vi "DWDT Digital to Binary U32.vi"(8 "error in (no error)":errorcluster, 11 "digital waveform":digitalwaveform(waveform)) -> (0 "error out":errorcluster, 3 "binary array":u32[](array[numeric]))   [LabVIEW 2020]
doc: "Converts a digital waveform or set of digital data to a binary array of unsigned integers. You must manually select the polymorphic instance you want to use."
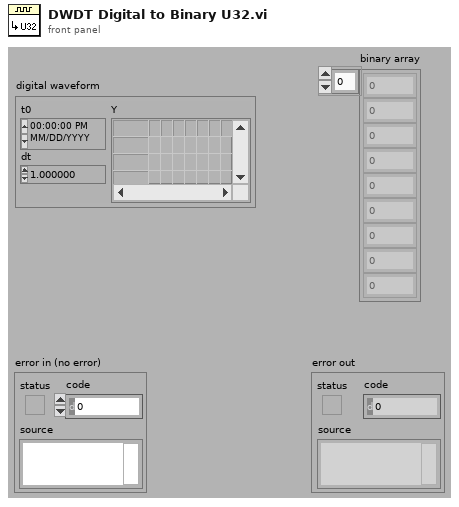
[diagram p1: front panel]
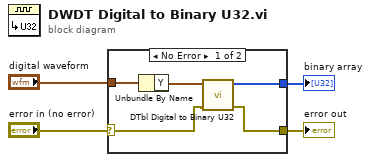
[diagram p0: block diagram]
diagram:
  n1 = case shown="No Error" "error in (no error)" {
    selector: "error in (no error)" -> [w6 w10]
    tunnel: [w5 w10] -> w3
    tunnel: "digital waveform" -> [w9 _]
    tunnel: [w7 _] -> w1
    frame No Error {
      n2 = Unbundle By Name(w9) -> ("Y"=w8:digitaldata)
      n3 = call "DTbl Digital to Binary U32.vi"("error in (no error)"=w6, "digital data"=w8) -> ("error out"=w5:errorcluster, "binary array"=w7:u32[])  [unwired: 8 in]
    }
    frame Error {
    }
  }
  "binary array" <- w1
  "error out" <- w3
